vi "List to Array.vi"(8 "List (empty)":string, 11 "Separator (,)":string=",") -> (0 "Output Number Array":dbl[](array[numeric]) format="%.2f", 3 "Output String Array":string[](array[string]))   [LabVIEW 2017, in "Agilent 34970.lvlib"]
doc: "Given a List of strings separated by a Separator, this VI returns the List as a String Array. If the strings are numbers, a Number Array is also returned."
uses:
  <instrlib>/Agilent 34970/Agilent 34970.lvlib
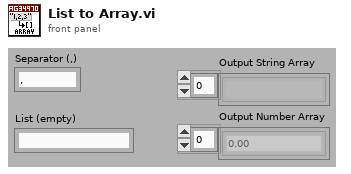
[diagram p1: front panel]
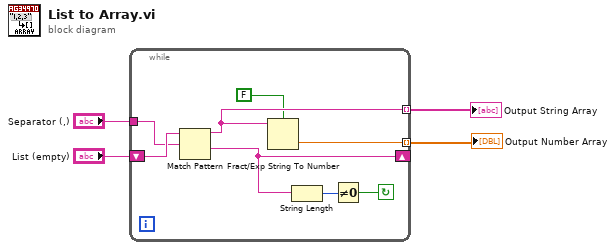
[diagram p0: block diagram]
diagram:
  n1 = while {
    tunnel: "Separator (,)" -> [w6]
    tunnel: [w7] -> w2 mode=indexing
    tunnel: [w9] -> w1 mode=indexing
    shift-left: "List (empty)" -> [w10]
    shift-right: [w8] -> _
    stop <- w12 continue-if-true
    n2 = Match Pattern(string=w10, regular expression=w6) -> (before substring=w7:string, after substring=w8:string)  [unwired: 1 in, 2 out]
    n3 = Fract/Exp String To Number(use system decimal point (T)=FALSE, string=w7) -> (number=w9:dbl)  [unwired: 2 in, 1 out]
    n4 = String Length(string=w8) -> (length=w11:i32)
    n5 = Not Equal To 0?(x=w11) -> (x != 0?=w12:bool)
  }
  "Output String Array" <- w2
  "Output Number Array" <- w1
